vi "CollisionAvoidanceEnabled_get.vi"(8 "error in (no error)":errorcluster) -> (0 "error out":errorcluster, 3 "Enabled":bool)   [LabVIEW 2009, in "Main.lvlib" / "MainVariables.lvlib"]
doc: "Get value of CollisionAvoidanceEnabled variable"
uses:
  MainVariables.lvlib
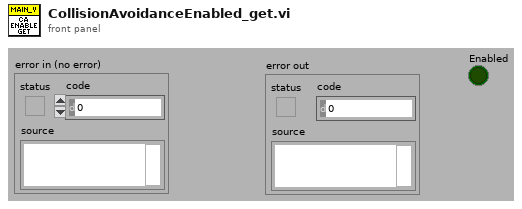
[diagram p1: front panel]
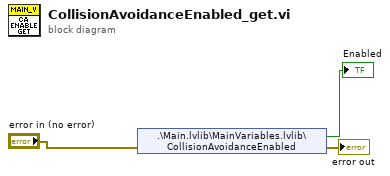
[diagram p0: block diagram]
diagram:
  n1 = shared-variable ".\\Main.lvlib\\MainVariables.lvlib\\CollisionAvoidanceEnabled"(error in="error in (no error)") -> (→"Enabled":bool, error out=→"error out":errorcluster)
